vi "Furnace_Control_2.vi"(6 "T Furnace":dbl, 7 "Counter Interval":i32, 8 "T Cat":dbl, 9 "T Set-Point":dbl, 10 "Furnace Set-point":dbl, 11 "Counter In":i32) -> (2 "Furnace Set-point":dbl, 3 "Counter Out":i32)   [LabVIEW 2014]
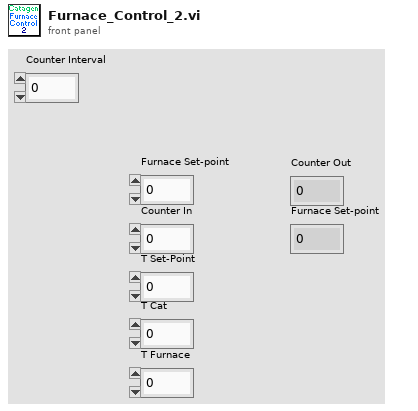
[diagram p1: front panel]
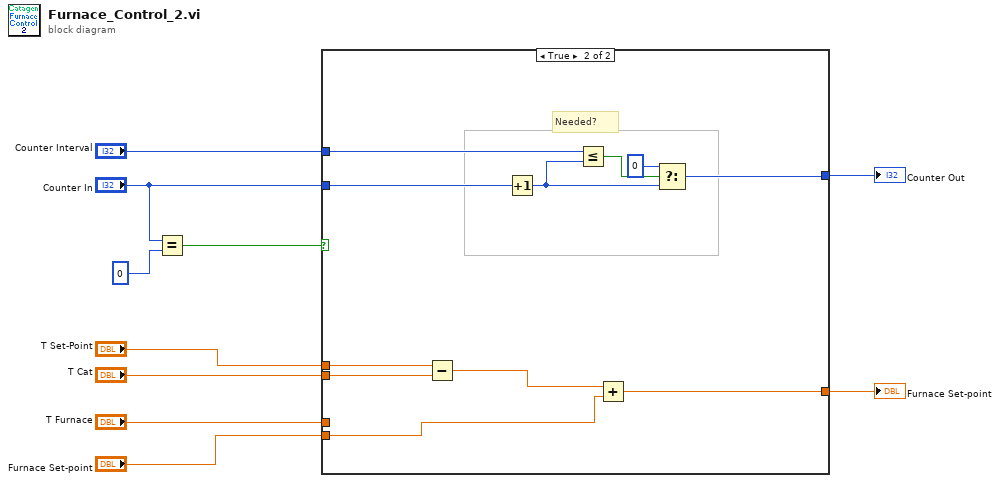
[diagram p0: block diagram]
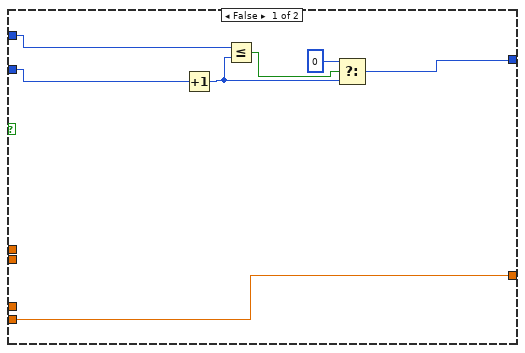
[diagram p2: hidden frame]
diagram:
  n1 = Equal?(x="Counter In", y=0) -> (x = y?=w10:bool)
  n2 = case shown="True" w10 {
    tunnel: "Counter In" -> [w13 w25]
    tunnel: [w12 w24] -> w4
    tunnel: "T Set-Point" -> [_ w28]
    tunnel: "T Cat" -> [_ w27]
    tunnel: "T Furnace" -> [_ _]
    tunnel: [w17 w26] -> w5
    tunnel: "Furnace Set-point" -> [w17 w18]
    tunnel: "Counter Interval" -> [w11 w20]
    frame False {
      n3 = Increment(x=w13) -> (x+1=w15:i32)
      n4 = Less Or Equal?(x=w11, y=w15) -> (x <= y?=w14:bool)
      n5 = Select(t=0, s=w14, f=w15) -> (s? t:f=w12:i32)
    }
    frame True {
      # "Needed?"
      n6 = Subtract(x=w28, y=w27) -> (x-y=w19:dbl)
      n7 = Increment(x=w25) -> (x+1=w22:i32)
      n8 = Less Or Equal?(x=w20, y=w22) -> (x <= y?=w21:bool)
      n9 = Add(x=w19, y=w18) -> (x+y=w26:dbl)
      n10 = Select(t=0, s=w21, f=w22) -> (s? t:f=w24:i32)
    }
  }
  "Furnace Set-point" <- w5
  "Counter Out" <- w4
